vi "PRBS9.vi"(1 "Size (Octets)":i32=37) -> (0 "Byte Array":u8[](array[numeric]) format="%o")   [LabVIEW 2013]
doc: "This vi will generate a Pseudorandom binary sequence based on a randomly generated seed. It uses the PRBS9 Polynomial, PRBS9 = x^{9} + x^{8} + 1"
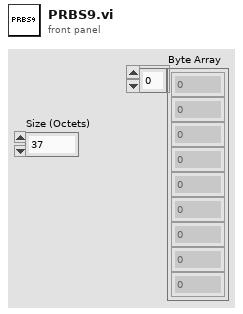
[diagram p1: front panel]
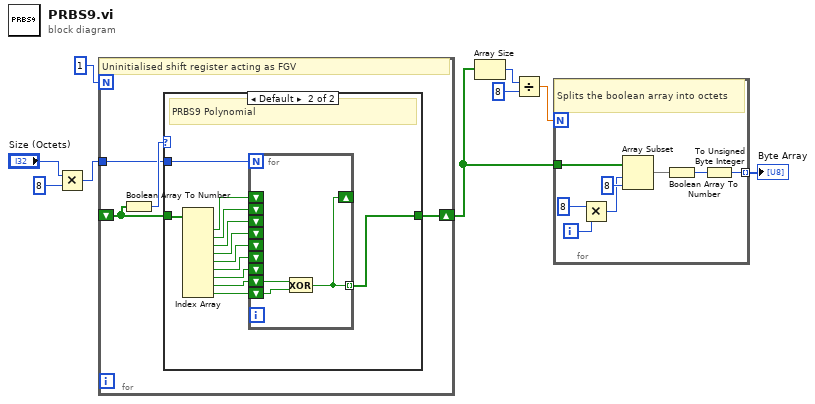
[diagram p0: block diagram]
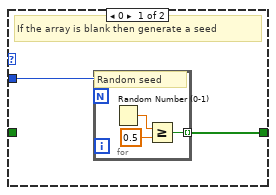
[diagram p2: hidden frame]
diagram:
  n1 = Multiply(x="Size (Octets)", y=8) -> (x*y=w6:i32)
  n2 = for {
    N: 1 -> [_]
    shift-right: [w13] -> w3
    shift-left: _ -> [w12]
    tunnel: w6 -> [w10]
    # "Uninitialised shift register acting as FGV"
    n3 = Boolean Array To Number(Boolean array=w12) -> (number=w11:u32)
    n4 = case shown="Default" w11 {
      tunnel: [w14 w21] -> w13
      tunnel: w12 -> [_ w20]
      tunnel: w10 -> [w15 w19]
      frame 0 {
        # "If the array is blank then generate a seed"
        n5 = for {
          N: w15 -> [_]
          tunnel: [w16] -> w14 mode=indexing
          # "Random seed"
          n6 = Random Number (0-1)() -> (number: 0 to 1=w18:dbl)
          n7 = Greater Or Equal?(x=w18, y=0.5) -> (x >= y?=w16:bool)
        }
      }
      frame Default {
        # "PRBS9 Polynomial"
        n8 = Index Array(array=w20) -> (element #1=w30:bool, element #2=w29:bool, element #3=w28:bool, element #4=w27:bool, element #5=w26:bool, element #6=w25:bool, element #7=w24:bool, element #8=w23:bool, element #9=w22:bool)  [unwired: 9 in]
        n9 = for {
          N: w19 -> [_]
          shift-right: [w31] -> _
          shift-left: w30 -> [_]
          shift-left: w29 -> [_]
          shift-left: w28 -> [_]
          shift-left: w27 -> [_]
          shift-left: w26 -> [_]
          shift-left: w25 -> [_]
          shift-left: w24 -> [_]
          shift-left: w23 -> [w32]
          shift-left: w22 -> [w33]
          tunnel: [w31] -> w21 mode=indexing
          n10 = Exclusive Or(1:w33, 2:w32) -> (0:w31:bool)
        }
      }
    }
  }
  n11 = Array Size(array=w3) -> (size(s)=w5:i32)
  n12 = Divide(x=w5, y=8) -> (x/y=w2:dbl)
  n13 = for {
    N: w2 -> [_]
    tunnel: w3 -> [w41]
    tunnel: [w34] -> w1 mode=indexing
    i -> [w39]
    # "Splits the boolean array into octets"
    n14 = Multiply(x=8, y=w39) -> (x*y=w37:i32)
    n15 = Array Subset(array=w41, index=w37, length=8) -> (w36:bool[])
    n16 = Boolean Array To Number(Boolean array=w36) -> (number=w35:u32)
    n17 = To Unsigned Byte Integer(number=w35) -> (unsigned 8bit integer=w34:u8)
  }
  "Byte Array" <- w1
